vi "Event Handler.vi"(0 "Guardian Subpanel in":refnum<class "Guardian Subpanel.lvclass">, 5 "Event type":T1=enum."Message", 7 "Item Name":string, 9 "Data":variant, 11 "error in (no error)":errorcluster) -> (4 "Guardian Subpanel out":refnum<class "Guardian Subpanel.lvclass">, 15 "error out":errorcluster)   [LabVIEW 2026, in "TALOS.lvlib" / "Guardian Subpanel.lvlib" / "Guardian Subpanel.lvclass"]
uses:
  Guardian Subpanel.lvclass
  C:/LabVIEW Code/TALOS/builds/Actor Framework PPL/Actor Framework.lvlibp/1abvi3w/vi.lib/ActorFramework/Actor/Actor.lvclass
  C:/LabVIEW Code/TALOS/talos/Father of all uServices/Father of all uServices/Father of all uServices.lvclass
  Father of all uServices/Father of all uServices/Event Handler Items.ctl
  Guardian/Guardian/Buttons_UI.ctl
  Guardian/Guardian Messages/Button Pressed Msg/Button Pressed Msg.lvclass/Button Pressed Msg.ctl
  Ancestor/Ancestor/Ancestor.lvclass/Ancestor.ctl
  Launch uService Message.ctl
  Guardian Subpanel Consumer Case Selector.ctl
  Father of all uServices/Father of all uServices Messages/Consumer Msg/Consumer Msg.lvclass/Consumer Msg.ctl
  Guardian/Guardian Messages/Message to uService Msg/Message to uService Msg.lvclass/Message to uService Msg.ctl
  Father of all uServices/Father of all uServices/Father of all uServices.lvclass/Father of all uServices.ctl
  <vilib>/Utility/error.llb/Trim Whitespace (string).vi
  FGV/Error Memory/Get Error Description.vi
  Support VIs/Get PC name.vi
  Ancestor/Ancestor/Read ID.vi
  Support VIs/Get Class Name.vi
  <vilib>/Utility/error.llb/Clear Errors.vi
  <vilib>/Utility/error.llb/Trim Whitespace One-Sided.vi
  Father of all uServices/Father of all uServices Messages/Consumer Msg/Send Consumer.vi
  Guardian/Guardian Messages/Message to uService Msg/Send Message to uService.vi
  Father of all uServices/Father of all uServices/Children Methods/Update GUI.vi
  FGV/Error Memory/Error Memory Core.vi
  <vilib>/AdvancedString/Delimited String to 1D String Array.vi
  <vilib>/AdvancedString/Delimited String to 1D String Array (string).vi
  Support VIs/Circus Root Path.vi
  FGV/Error Memory/Error Crt Lvl checker.vi
  FGV/Error Memory/Error Memory Core.vi/40c8088d-b597-4017-91af-faa98e00292e.vi
  FGV/Error Memory/Error Memory Core.vi/d4a3ab98-063c-4e44-b43d-fbdcfe6c2be2.vi
  Father of all uServices/Father of all uServices/Father of all uServices.lvclass
  builds/Actor Framework PPL/Actor Framework.lvlibp/1abvi3w/vi.lib/ActorFramework/Message Enqueuer/Enqueue.vi
  Support VIs/Global Memory.vi
  <vilib>/Utility/LVClass/Get LV Class Name.vi
  Support VIs/Is in Packed Library.vi
  Support VIs/TALOS Root path.vi
  Support VIs/Read CSV worksheet.vi
  Support VIs/Global Constants.vi
  <vilib>/Utility/error.llb/General Error Handler.vi
  Update Git Confirmation Window.vi
  Support VIs/Error Log.vi
  builds/Actor Framework PPL/Actor Framework.lvlibp/1abvi3w/vi.lib/ActorFramework/Actor/Read Self Enqueuer.vi
  <userlib>/_OpenG.lib/lvdata/lvdata.llb/Get Strings from Enum__ogtk.vi
  Father of all uServices/Father of all uServices/Multiline string updater.vi
  Guardian/Guardian Messages/Button Pressed Msg/Button Pressed Msg.lvclass
  Ancestor/Ancestor/Ancestor.lvclass
  <vilib>/Comparison/Equal/Equal Functor/Equal Functor.lvclass
  Father of all uServices/Father of all uServices Messages/Consumer Msg/Consumer Msg.lvclass
  Guardian/Guardian Messages/Message to uService Msg/Message to uService Msg.lvclass
  TALOS.lvlib
  Guardian/Guardian/Guardian.lvclass
  builds/Actor Framework PPL/Actor Framework.lvlibp/1abvi3w/vi.lib/ActorFramework/Actor/Actor.lvclass
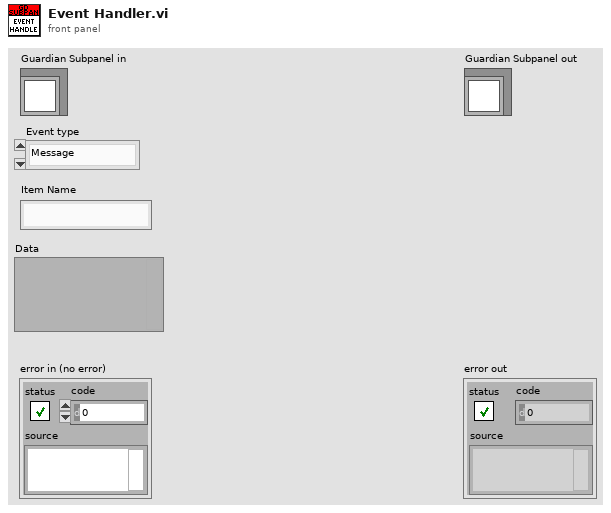
[diagram p1: front panel]
types:
  T1 = typedef "TALOS.lvlib/Father of all uServices.lvlib/Father of all uServices.lvclass/Event Handler Items.ctl" = enum16{"Button Pressed", "Message", "Ready to launch?", "Safe Mode", "Start RUN", "Stop RUN"}
  T2 = typedef "TALOS.lvlib/Guardian.lvlib/Guardian.lvclass/Buttons_UI.ctl" = enum16{"Start uService", "Kill uService", "Stop uService", "Stop", "Start online checks", "Stop online checks", "Send Pat to all GDs", "Reload INI files", "Update from GIT", "RUN", "Reset ABORT", "Check Bearer", "Send I Exist", "Change Run Config", "Add uSs from Config", "Realign uSs from Config", "Send Run Config to GD"}
  T3 = typedef "TALOS.lvlib/Guardian Subpanel.lvlib/Guardian Subpanel.lvclass/Launch uService Message.ctl" = cluster{"uService Class Name":string, "uService ID":string}
  T4 = typedef "TALOS.lvlib/Guardian Subpanel.lvlib/Guardian Subpanel.lvclass/Guardian Subpanel Consumer Case Selector.ctl" = enum16{"uServices launchable", "Update Bearer"}
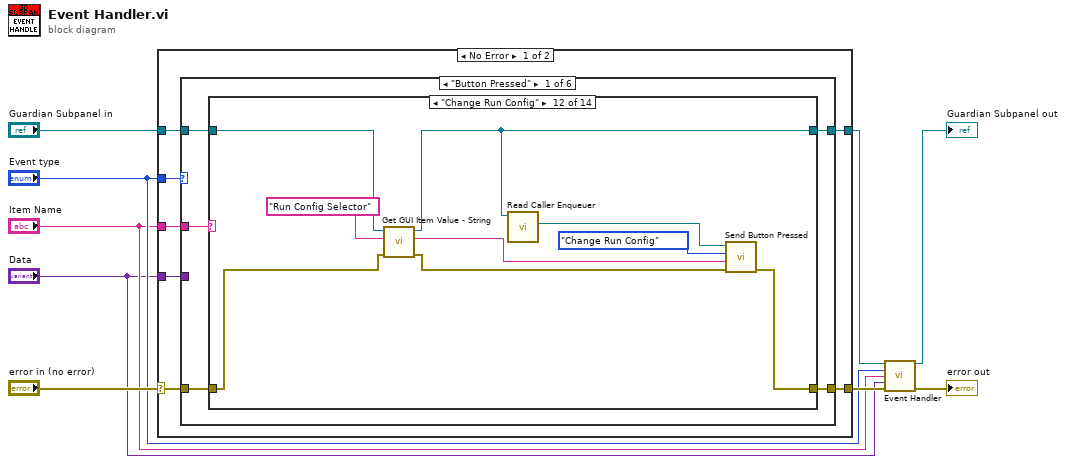
[diagram p0: block diagram]
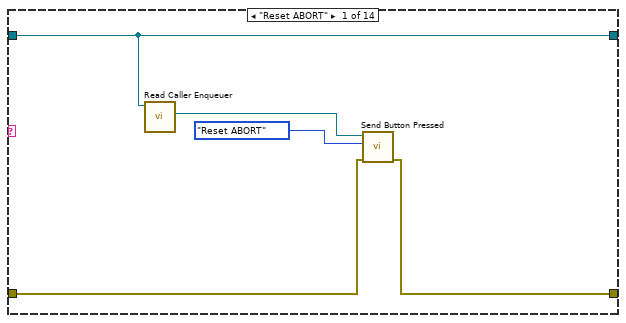
[diagram p2: hidden frame]
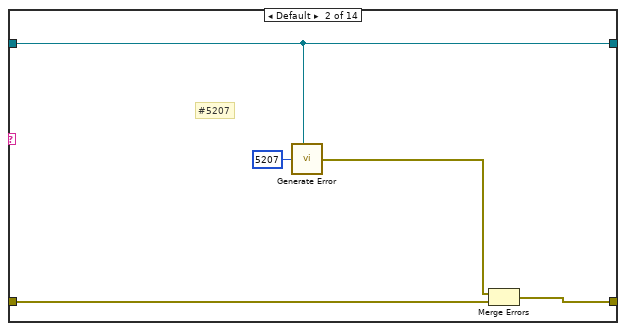
[diagram p3: hidden frame]
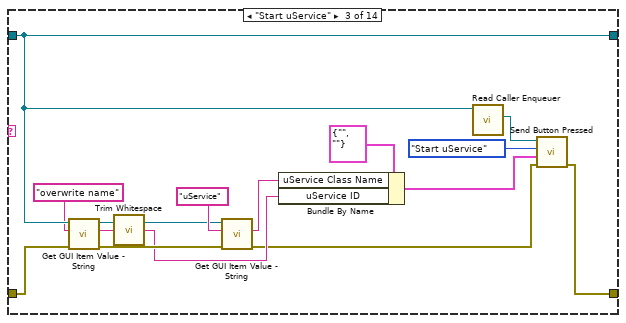
[diagram p4: hidden frame]
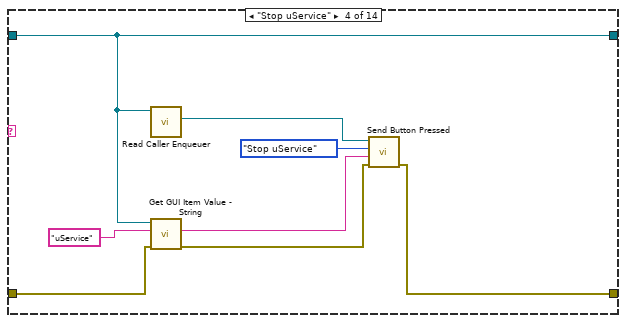
[diagram p5: hidden frame]
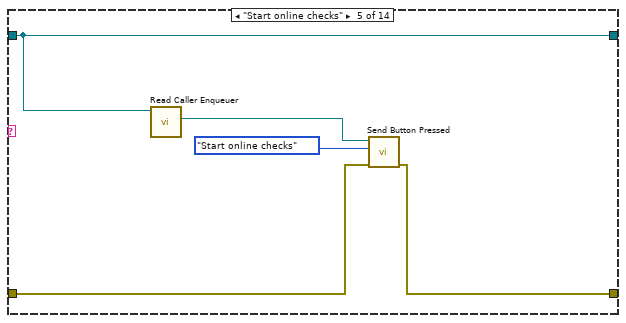
[diagram p6: hidden frame]
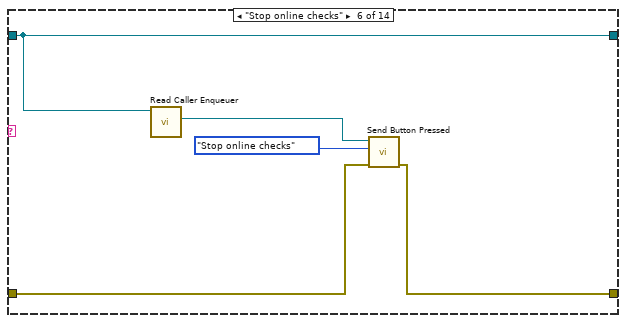
[diagram p7: hidden frame]
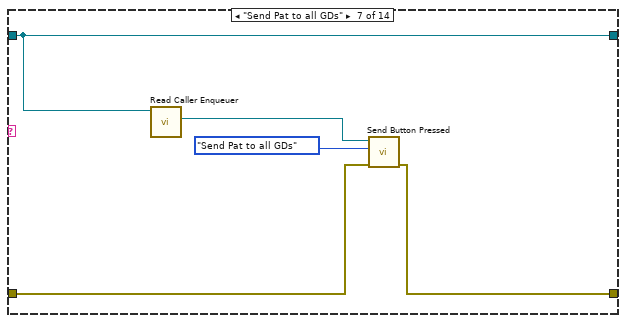
[diagram p8: hidden frame]
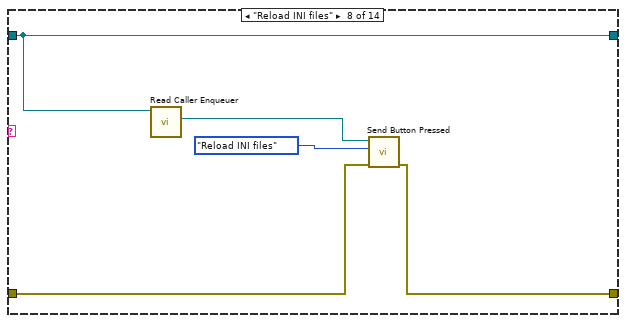
[diagram p9: hidden frame]
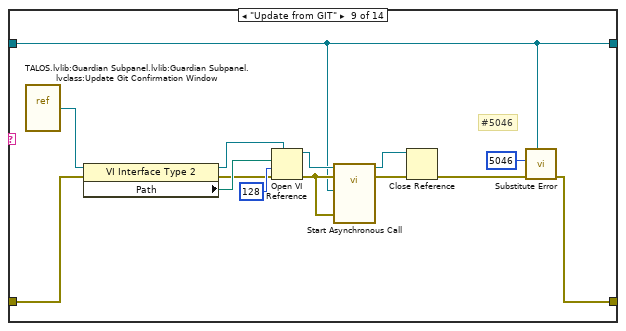
[diagram p10: hidden frame]
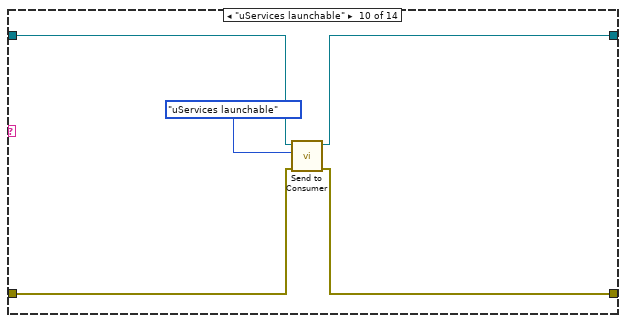
[diagram p11: hidden frame]
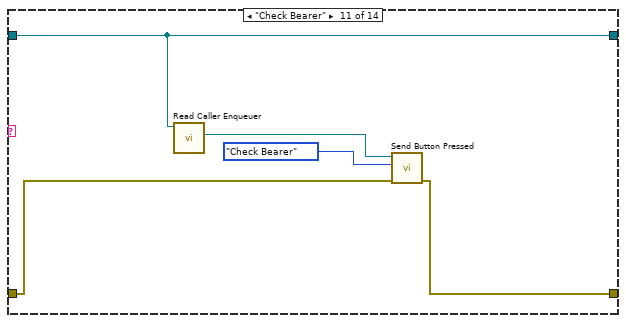
[diagram p12: hidden frame]
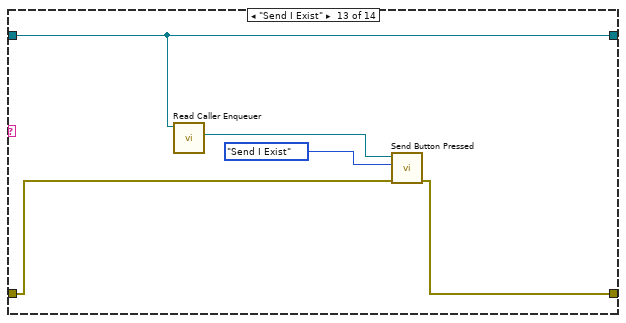
[diagram p13: hidden frame]
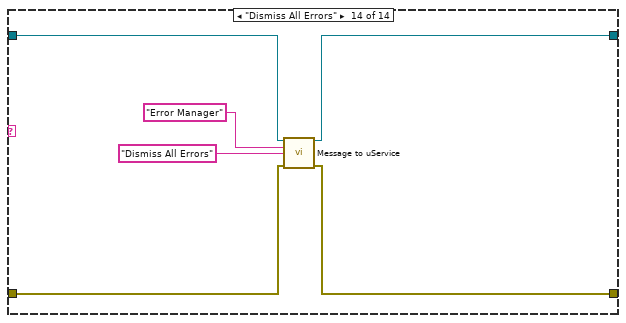
[diagram p14: hidden frame]
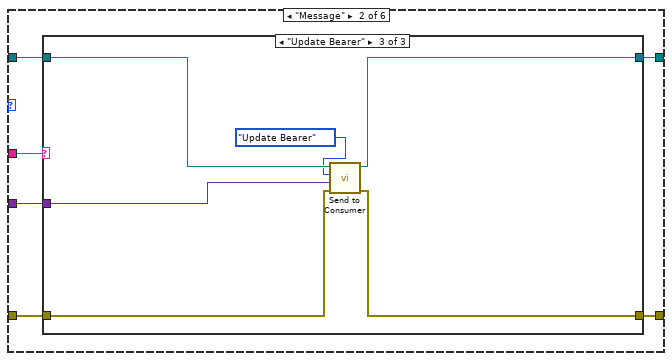
[diagram p15: hidden frame]
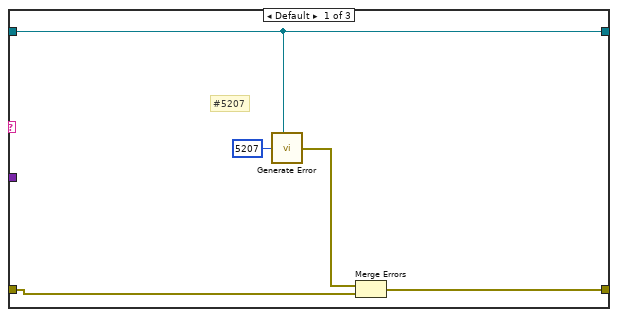
[diagram p16: hidden frame]
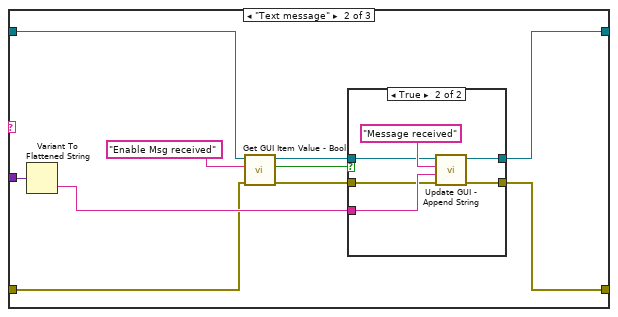
[diagram p17: hidden frame]
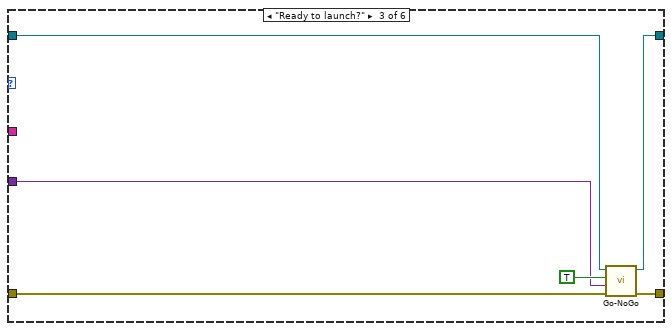
[diagram p19: hidden frame]
diagram:
  n1 = case shown="No Error" "error in (no error)" {
    selector: "error in (no error)" -> [w13 w167]
    tunnel: [w12 w167] -> w7
    tunnel: "Guardian Subpanel in" -> [w15 w166]
    tunnel: [w14 w166] -> w4
    tunnel: "Event type" -> [w16 _]
    tunnel: "Item Name" -> [w11 _]
    tunnel: "Data" -> [w10 _]
    frame No Error {
      n2 = case shown="\"Button Pressed\"" w16 {
        tunnel: w15 -> [w21 w124 w156 w161 w163 w165]
        tunnel: [w20 w120 w159 w161 w163 w165] -> w14
        tunnel: w13 -> [w17 w121 w157 w160 w162 w164]
        tunnel: [w18 w119 w158 w160 w162 w164] -> w12
        tunnel: w11 -> [w19 w123 _ _ _ _]
        tunnel: w10 -> [_ w122 w154 _ _ _]
        frame "Button Pressed" {
          n3 = case shown="\"Change Run Config\"" w19 {
            tunnel: w21 -> [w24 w27 w43 w47 w55 w60 w65 w70 w77 w92 w96 w100 w110 w114]
            tunnel: [w24 w27 w43 w47 w55 w60 w65 w70 w77 w93 w96 w101 w110 w113] -> w20
            tunnel: [w23 w30 w44 w48 w56 w61 w66 w71 w78 w90 w94 w105 w108 w115] -> w18
            tunnel: w17 -> [w22 w31 w41 w50 w57 w62 w67 w72 w80 w91 w95 w102 w109 w116]
            frame "Reset ABORT" {
              n4 = call "Read Caller Enqueuer.vi"("Actor"=w24) -> ("Caller Enqueuer"=w25:refnum<class "Message Enqueuer.lvclass">)  [unwired: 10 in]
              n5 = call "Send Button Pressed.vi"("error in (no error)"=w22, "Button"=Buttons_UI."Reset ABORT", "Message Enqueuer"=w25) -> ("error out"=w23:errorcluster)  [unwired: 7 in, 1 out]
            }
            frame Default {
              # "#5207"
              n6 = call "Generate Error.vi"("Class"=w27, "Error Code"=5207) -> ("error out"=w29:errorcluster)  [unwired: 5 in]
              n7 = Merge Errors(w29, w31) -> (w30:errorcluster)
            }
            frame "Start uService" {
              n8 = call "Get GUI Item Value - String.vi"("error in (no error)"=w41, "FP Item Name"="overwrite name", "uService Template in"=w43) -> ("error out"=w38:errorcluster, "Value"=w42:string, "uService Template out"=w39:refnum<class "Guardian Subpanel.lvclass">)  [unwired: 6 in]
              n9 = call-poly <vilib>:"Trim Whitespace.vi"("string"=w42) -> ("trimmed string"=w35:string)  [unwired: 1 in]
              n10 = call "Get GUI Item Value - String.vi"("error in (no error)"=w38, "FP Item Name"="uService", "uService Template in"=w39) -> ("error out"=w33:errorcluster, "Value"=w36:string)  [unwired: 6 in, 1 out]
              n11 = Bundle By Name(cluster=T3 {"uService Class Name"="", "uService ID"=""} ("Cluster"), "uService Class Name"=w36, "uService ID"=w35) -> (w34:T3)
              n12 = call "Read Caller Enqueuer.vi"("Actor"=w43) -> ("Caller Enqueuer"=w45:refnum<class "Message Enqueuer.lvclass">)  [unwired: 10 in]
              n13 = call "Send Button Pressed.vi"("error in (no error)"=w33, "Data"=w34, "Button"=Buttons_UI."Start uService", "Message Enqueuer"=w45) -> ("error out"=w44:errorcluster)  [unwired: 6 in, 1 out]
            }
            frame "Stop uService" {
              n14 = call "Read Caller Enqueuer.vi"("Actor"=w47) -> ("Caller Enqueuer"=w52:refnum<class "Message Enqueuer.lvclass">)  [unwired: 10 in]
              n15 = call "Get GUI Item Value - String.vi"("error in (no error)"=w50, "FP Item Name"="uService", "uService Template in"=w47) -> ("error out"=w49:errorcluster, "Value"=w51:string)  [unwired: 6 in, 1 out]
              n16 = call "Send Button Pressed.vi"("error in (no error)"=w49, "Data"=w51, "Button"=Buttons_UI."Stop uService", "Message Enqueuer"=w52) -> ("error out"=w48:errorcluster)  [unwired: 6 in, 1 out]
            }
            frame "Start online checks" {
              n17 = call "Read Caller Enqueuer.vi"("Actor"=w55) -> ("Caller Enqueuer"=w58:refnum<class "Message Enqueuer.lvclass">)  [unwired: 10 in]
              n18 = call "Send Button Pressed.vi"("error in (no error)"=w57, "Button"=Buttons_UI."Start online checks", "Message Enqueuer"=w58) -> ("error out"=w56:errorcluster)  [unwired: 7 in, 1 out]
            }
            frame "Stop online checks" {
              n19 = call "Read Caller Enqueuer.vi"("Actor"=w60) -> ("Caller Enqueuer"=w63:refnum<class "Message Enqueuer.lvclass">)  [unwired: 10 in]
              n20 = call "Send Button Pressed.vi"("error in (no error)"=w62, "Button"=Buttons_UI."Stop online checks", "Message Enqueuer"=w63) -> ("error out"=w61:errorcluster)  [unwired: 7 in, 1 out]
            }
            frame "Send Pat to all GDs" {
              n21 = call "Read Caller Enqueuer.vi"("Actor"=w65) -> ("Caller Enqueuer"=w68:refnum<class "Message Enqueuer.lvclass">)  [unwired: 10 in]
              n22 = call "Send Button Pressed.vi"("error in (no error)"=w67, "Button"=Buttons_UI."Send Pat to all GDs", "Message Enqueuer"=w68) -> ("error out"=w66:errorcluster)  [unwired: 7 in, 1 out]
            }
            frame "Reload INI files" {
              n23 = call "Read Caller Enqueuer.vi"("Actor"=w70) -> ("Caller Enqueuer"=w73:refnum<class "Message Enqueuer.lvclass">)  [unwired: 10 in]
              n24 = call "Send Button Pressed.vi"("error in (no error)"=w72, "Button"=Buttons_UI."Reload INI files", "Message Enqueuer"=w73) -> ("error out"=w71:errorcluster)  [unwired: 7 in, 1 out]
            }
            frame "Update from GIT" {
              # "#5046"
              n25 = vi-ref "TALOS.lvlib:Guardian Subpanel.lvlib:Guardian Subpanel.lvclass:Update Git Confirmation Window.vi"() -> (w75:refnum<vi>)
              n26 = property class="VI Interface Type 2"(reference=w75, error in=w80) -> (reference out=w84:refnum<vi>, error out=w82:errorcluster, "Path"=w83:path)
              n27 = Open VI Reference(type specifier VI Refnum (for type only)=w84, vi path=w83, options=128, error in (no error)=w82) -> (vi reference=w88:refnum<vi>, error out=w81:errorcluster)  [unwired: 2 in]
              n28 = call-by-ref "Start Asynchronous Call"(reference=w88, error in=w81, 8:"error in (no error)"=w81, "Guardian Subpanel in"=w77) -> (reference out=w86:refnum<vi>, error out=w87:errorcluster)  [unwired: 9 in, 1 out]
              n29 = Close Reference(reference=w86, error in (no error)=w87) -> (error out=w79:errorcluster)
              n30 = call "Substitute Error.vi"("LabVIEW Object"=w77, "error in (no error)"=w79, "Error Code"=5046) -> ("error out"=w78:errorcluster)  [unwired: 8 in]
            }
            frame "uServices launchable" {
              n31 = call "Send to Consumer.vi"("error in (no error)"=w91, "Case ID"=Guardian_Subpanel_Consumer_Case_Selector."uServices launchable" ("Guardian Subpanel Consumer Case Selector"), "uService Template in"=w92) -> ("error out"=w90:errorcluster, "uService Template out"=w93:refnum<class "Guardian Subpanel.lvclass">)  [unwired: 7 in]
            }
            frame "Check Bearer" {
              n32 = call "Read Caller Enqueuer.vi"("Actor"=w96) -> ("Caller Enqueuer"=w97:refnum<class "Message Enqueuer.lvclass">)  [unwired: 10 in]
              n33 = call "Send Button Pressed.vi"("error in (no error)"=w95, "Button"=Buttons_UI."Check Bearer", "Message Enqueuer"=w97) -> ("error out"=w94:errorcluster)  [unwired: 7 in, 1 out]
            }
            frame "Change Run Config" {
              n34 = call "Get GUI Item Value - String.vi"("error in (no error)"=w102, "FP Item Name"="Run Config Selector", "uService Template in"=w100) -> ("error out"=w103:errorcluster, "Value"=w99:string, "uService Template out"=w101:refnum<class "Guardian Subpanel.lvclass">)  [unwired: 6 in]
              n35 = call "Read Caller Enqueuer.vi"("Actor"=w101) -> ("Caller Enqueuer"=w106:refnum<class "Message Enqueuer.lvclass">)  [unwired: 10 in]
              n36 = call "Send Button Pressed.vi"("error in (no error)"=w103, "Data"=w99, "Button"=Buttons_UI."Change Run Config", "Message Enqueuer"=w106) -> ("error out"=w105:errorcluster)  [unwired: 6 in, 1 out]
            }
            frame "Send I Exist" {
              n37 = call "Read Caller Enqueuer.vi"("Actor"=w110) -> ("Caller Enqueuer"=w111:refnum<class "Message Enqueuer.lvclass">)  [unwired: 10 in]
              n38 = call "Send Button Pressed.vi"("error in (no error)"=w109, "Button"=Buttons_UI."Send I Exist", "Message Enqueuer"=w111) -> ("error out"=w108:errorcluster)  [unwired: 7 in, 1 out]
            }
            frame "Dismiss All Errors" {
              n39 = call "Message to uService.vi"("Father of all uServices in"=w114, "uService ID"="Error Manager", "Message"="Dismiss All Errors", "error in (no error)"=w116) -> ("Father of all uServices out"=w113:refnum<class "Guardian Subpanel.lvclass">, "error out"=w115:errorcluster)  [unwired: 10 in]
            }
          }
        }
        frame "Message" {
          n40 = case shown="\"Update Bearer\"" w123 {
            tunnel: w124 -> [w127 w132 w153]
            tunnel: w122 -> [_ w139 w151]
            tunnel: w121 -> [w125 w134 w150]
            tunnel: [w127 w138 w148] -> w120
            tunnel: [w126 w137 w149] -> w119
            frame Default {
              # "#5207"
              n41 = call "Generate Error.vi"("Class"=w127, "Error Code"=5207) -> ("error out"=w128:errorcluster)  [unwired: 5 in]
              n42 = Merge Errors(w128, w125) -> (w126:errorcluster)
            }
            frame "Text message" {
              n43 = Variant To Flattened String(Variant=w139) -> (data string=w135:string)  [unwired: 1 out]
              n44 = call "Get GUI Item Value - Bool.vi"("error in (no error)"=w134, "FP Item Name"="Enable Msg received", "uService Template in"=w132) -> ("error out"=w133:errorcluster, "Value"=w130:bool, "uService Template out"=w131:refnum<class "Guardian Subpanel.lvclass">)  [unwired: 6 in]
              n45 = case shown="True" w130 {
                tunnel: [w141 w146] -> w138
                tunnel: [w140 w145] -> w137
                tunnel: w135 -> [_ w144]
                tunnel: w133 -> [w140 w143]
                tunnel: w131 -> [w141 w142]
                frame False {
                }
                frame True {
                  n46 = call "Update GUI - Append String.vi"("error in (no error)"=w143, "String"=w144, "GUI Item Name"="Message received", "Father of all uServices in"=w142) -> ("error out"=w145:errorcluster, "Father of all uServices out"=w146:refnum<class "Guardian Subpanel.lvclass">)  [unwired: 6 in]
                }
              }
            }
            frame "Update Bearer" {
              n47 = call "Send to Consumer.vi"("error in (no error)"=w150, "Data"=w151, "Case ID"=Guardian_Subpanel_Consumer_Case_Selector."Update Bearer" ("Guardian Subpanel Consumer Case Selector"), "uService Template in"=w153) -> ("error out"=w149:errorcluster, "uService Template out"=w148:refnum<class "Guardian Subpanel.lvclass">)  [unwired: 6 in]
            }
          }
        }
        frame "Ready to launch?" {
          n48 = call-dynamic "Go-NoGo.vi"("error in (no error)"=w157, "Go-NoGo Data"=w154, "Go?"=TRUE, "Father of all uServices in"=w156) -> ("error out"=w158:errorcluster, "Father of all uServices out"=w159:refnum<class "Guardian Subpanel.lvclass">)  [unwired: 6 in]
        }
        frame "Safe Mode" {
        }
        frame "Start RUN" {
        }
        frame "Stop RUN" {
        }
      }
    }
    frame Error {
    }
  }
  n49 = call-parent "Event Handler.vi"("uService Template in"=w4, "Event type"="Event type", "Item Name"="Item Name", "Data"="Data", "error in (no error)"=w7) -> ("uService Template out"=→"Guardian Subpanel out":refnum<class "Guardian Subpanel.lvclass">, "error out"=→"error out":errorcluster)  [unwired: 9 in]
